vi "waveform history.vi"(10 "# periods":i32, 11 "Array":waveform(dbl)[](array[waveform])) -> (3 "Array 2":waveform(dbl)[](array[waveform]))   [LabVIEW 2013]
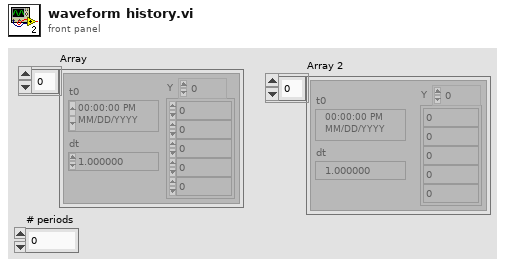
[diagram p1: front panel]
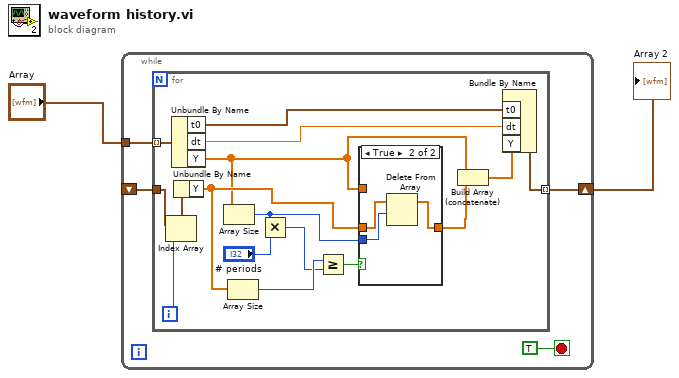
[diagram p0: block diagram]
diagram:
  n1 = while {
    shift-right: [w3] -> w2
    shift-left: _ -> [w4]
    tunnel: "Array" -> [w5]
    stop <- TRUE stop-if-true
    n2 = for {
      tunnel: w5 -> [w16] mode=indexing
      tunnel: w4 -> [w11]
      tunnel: [w15] -> w3 mode=indexing
      i -> [w12]
      n3 = Index Array(array=w11, index=w12) -> (element=w10:waveform(dbl))
      n4 = Unbundle By Name(w16) -> ("t0"=w14:timestamp, "dt"=w13:dbl, "Y"=w9:dbl[])
      n5 = Unbundle By Name(w10) -> ("Y"=w17:dbl[])
      n6 = Array Size(array=w9) -> (size(s)=w19:i32)
      n7 = Array Size(array=w17) -> (size(s)=w21:i32)
      n8 = Multiply(x=w19, y="# periods") -> (x*y=w20:i32)
      n9 = Greater Or Equal?(x=w21, y=w20) -> (x >= y?=w18:bool)
      n10 = case shown="True" w18 {
        tunnel: w19 -> [_ w25]
        tunnel: w17 -> [w23 w26]
        tunnel: [w23 w24] -> w7
        tunnel: w9 -> [_ _]
        frame False {
        }
        frame True {
          n11 = Delete From Array(array=w26, length=w25) -> (array with subset deleted=w24:dbl[])  [unwired: 1 in, 1 out]
        }
      }
      n12 = Build Array (concatenate)(w9, w7) -> (w8:dbl[])
      n13 = Bundle By Name("t0"=w14, "dt"=w13, "Y"=w8) -> (w15:waveform(dbl))  [unwired: 1 in]
    }
  }
  "Array 2" <- w2
